vi "Python Predict.vi"(4 "Piezo_Volts":dbl[](array[numeric]), 6 "tdms file":refnum<k34>, 7 "Array":sgl[](array[numeric]), 8 "error in (no error)":errorcluster, 9 "Array 2":sgl[](array[numeric]), 10 "module path":path, 11 "Refnum in":refnum<k35>) -> (0 "error out":errorcluster, 1 "piezo volt Pred":dbl, 3 "Cluster":cluster{"X Centroid":dbl, "X Centroid":dbl})   [LabVIEW 2020]
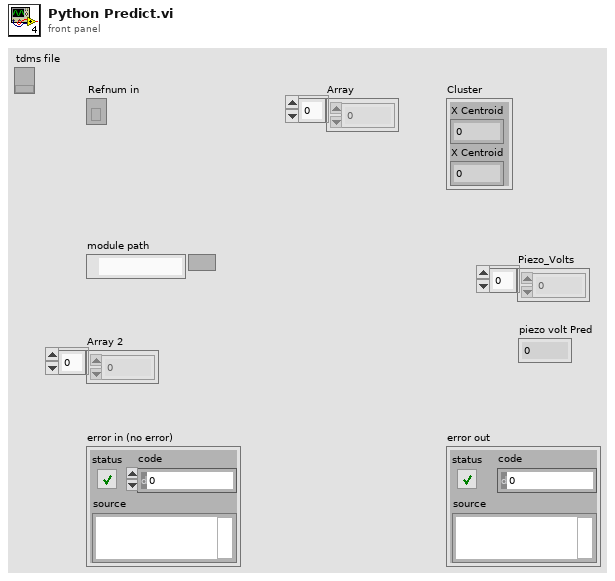
[diagram p1: front panel]
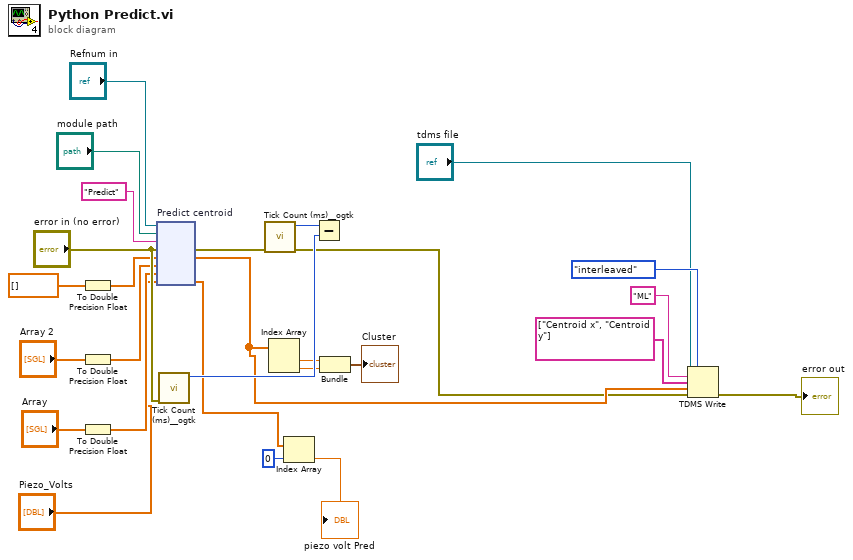
[diagram p0: block diagram]
diagram:
  n1 = To Double Precision Float(number=sgl[] []) -> (double precision float=w18:dbl[])
  n2 = To Double Precision Float(number="Array 2") -> (double precision float=w20:dbl[])
  n3 = To Double Precision Float(number="Array") -> (double precision float=w23:dbl[])
  n4 = node "Predict centroid"("Refnum in", "module path", "Predict" ("function name"), "error in (no error)", w18, w20, w23, "Piezo_Volts") -> (w24:errorcluster, w8:dbl[], w2:dbl[])  [unwired: 2 in, 3 out]
  n5 = call <userlib>:"Tick Count (ms)__ogtk.vi"("error in (no error)"="error in (no error)") -> ("millisecond timer value"=w27:u32)  [unwired: 9 in, 1 out]
  n6 = call <userlib>:"Tick Count (ms)__ogtk.vi"("error in (no error)"=w24) -> ("error out"=w6:errorcluster, "millisecond timer value"=w26:u32)  [unwired: 9 in]
  n7 = Index Array(array=w8) -> (element #1=w16:dbl, element #2=w15:dbl)  [unwired: 2 in]
  n8 = Index Array(array=w2, index=0) -> (element=→"piezo volt Pred":dbl)
  n9 = Subtract(x=w26, y=w27) -> ()  [unwired: 1 out]
  n10 = Bundle("X Centroid"=w16, "X Centroid"=w15) -> (→"Cluster":cluster{"X Centroid":dbl, "X Centroid":dbl})  [unwired: 1 in]
  n11 = TDMS Write(0:"tdms file", 1:enum16{"decimated", "interleaved"}."interleaved" ("data layout (0:decimated)"), 5:"ML" ("group name in (Untitled)"), 7:string[] ["Centroid x", "Centroid y"] ("channel name(s) in (Untitled)"), 9:w8, 11:w6) -> (15:→"error out":errorcluster)  [unwired: 3 out]
